vi "Smart Attacker.vi"(8 "error in (no error)":errorcluster, 10 "Map":i32[](array[numeric]), 11 "Mother In":refnum<class "Base Builder.lvclass">) -> (0 "error out":errorcluster, 1 "Direction":T1, 2 "Action":T2, 3 "Mother Out":refnum<class "Base Builder.lvclass">, 4 "Replicated":refnum<class "Square.lvclass">)   [LabVIEW 2015, in "Base Builder.lvclass"]
uses:
  Base Builder/Base Builder.lvclass
  Type Defs/Action Enum.ctl
  Type Defs/Direction Enum.ctl
  Square/Square.lvclass
  Base Builder/Base Builder.lvclass/Base Builder.ctl
  Formics/Attack Options.ctl
  Formics/Coward Options.ctl
  Common/Common.lvlib
  Formics/Formics.lvclass
  Type Defs/SB Type Defs.lvlib
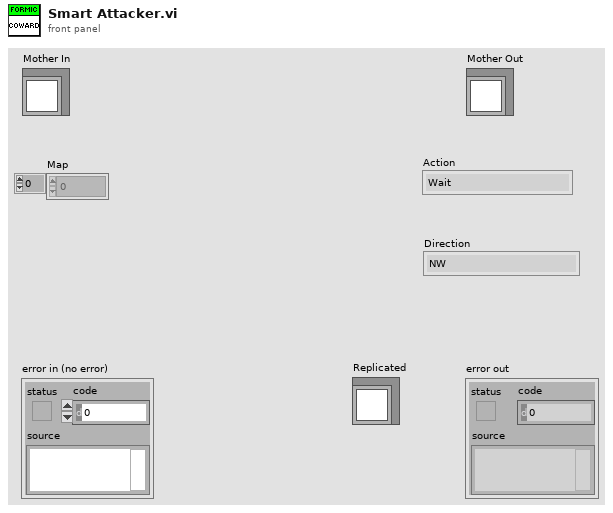
[diagram p1: front panel]
types:
  T1 = typedef "SB Type Defs.lvlib/Direction Enum.ctl" = enum16{"NW", "N", "NE", "E", "SE", "S", "SW", "W"}
  T2 = typedef "SB Type Defs.lvlib/Action Enum.ctl" = enum16{"Wait", "Move", "Attack", "Replicate"}
  T3 = typedef "Formics.lvclass/Coward Options.ctl" = enum16{"Go", "Attack behind and continue", "Attack behind and recheck", "Move Back", "Check if still there"}
  T4 = typedef "Formics.lvclass/Attack Options.ctl" = enum16{"Attack", "Run", "Distract"}
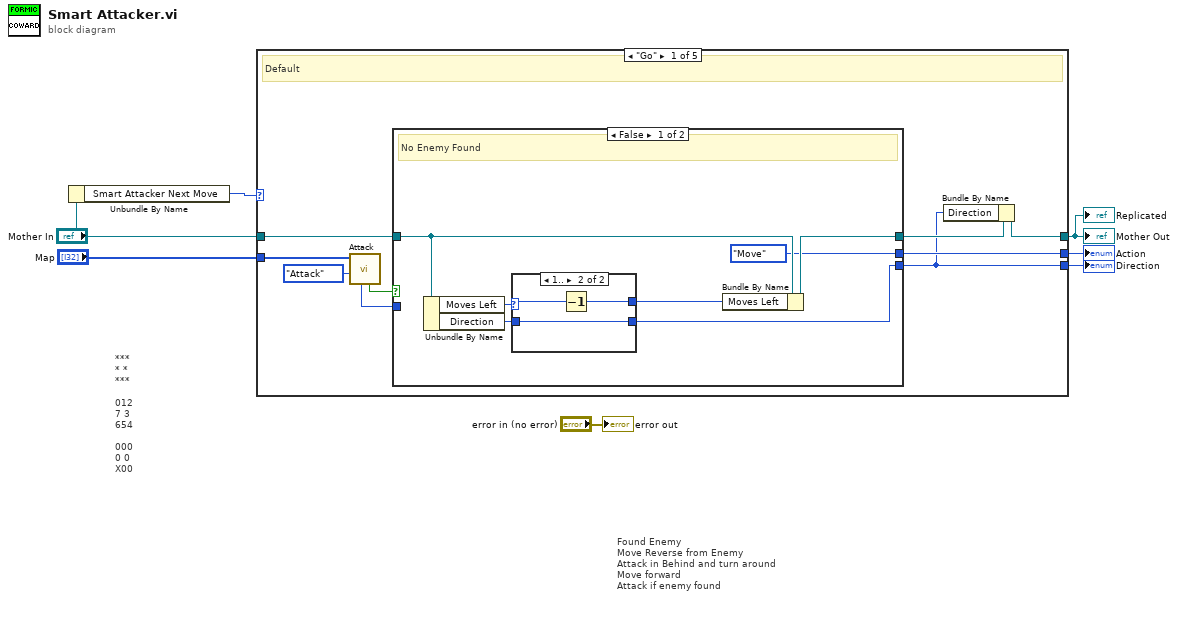
[diagram p0: block diagram]
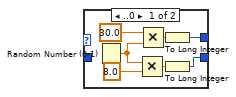
[diagram p2: hidden frame]
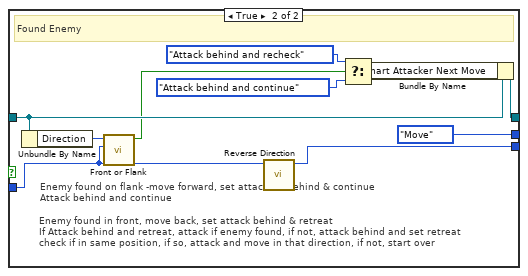
[diagram p3: hidden frame]
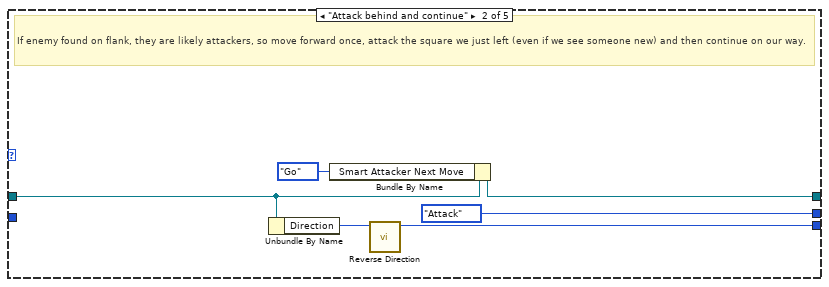
[diagram p4: hidden frame]
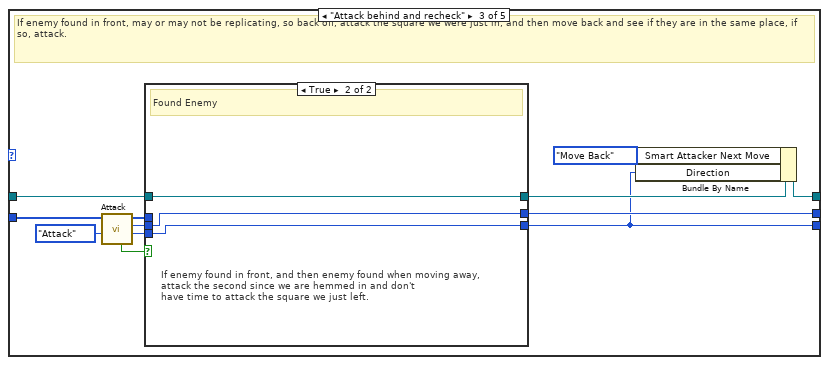
[diagram p5: hidden frame]
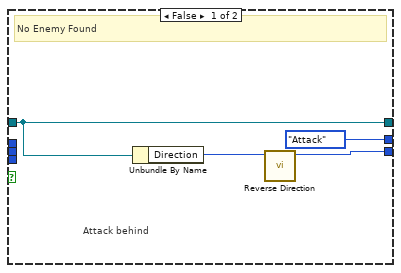
[diagram p6: hidden frame]
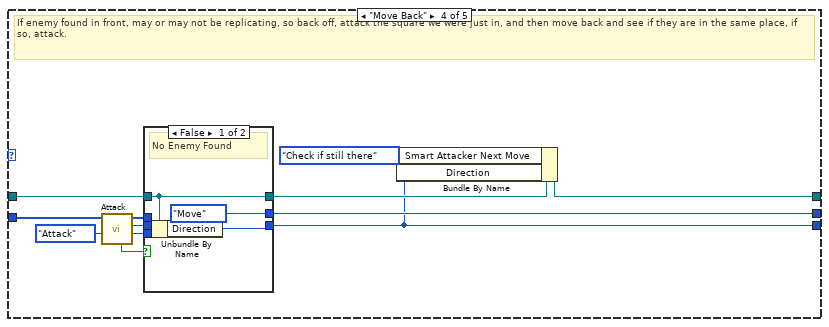
[diagram p7: hidden frame]
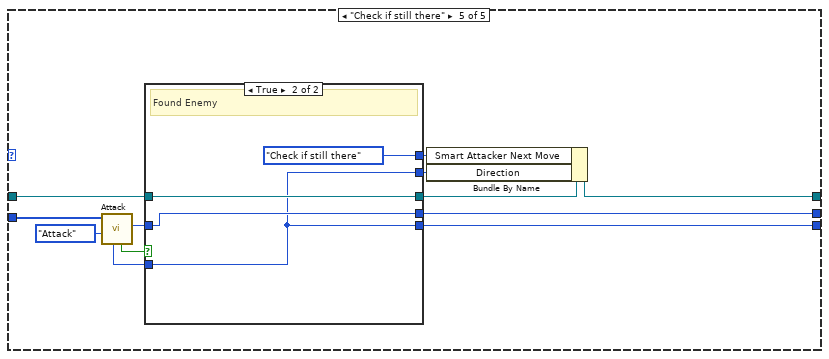
[diagram p9: hidden frame]
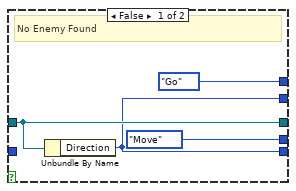
[diagram p10: hidden frame]
diagram:
  # "Found Enemy\nMove Reverse from Enemy\nAttack in Behind and turn around\nMove forward\nAttack if enemy found"
  # "***\n* *\n***\n\n012\n7 3\n654\n\n000\n0 0\nX00"
  n1 = Unbundle By Name("Mother In") -> ("Smart Attacker Next Move"=w2:T3)
  n2 = case shown="\"Go\"" w2 {
    tunnel: [w14 Action_Enum."Attack" ("Action") w58 w77 w95] -> w6
    tunnel: [w9 w48 w50 w69 w94] -> w5
    tunnel: [w10 w47 w52 w71 w90] -> w1
    tunnel: "Map" -> [w12 _ w54 w73 w92]
    tunnel: "Mother In" -> [w11 w44 w53 w72 w91]
    frame "Go" {
      # "Default"
      n3 = call "Attack.vi"("Attack?"=Attack_Options."Attack", "Maze (0: Empty, -1: Enemy. >0: Teammate"=w12) -> ("Enemy Found?"=w15:bool, "Enemy Direction"=w8:i32)  [unwired: 4 in, 4 out]
      n4 = case shown="False" w15 {
        tunnel: [Action_Enum."Move" ("Action") Action_Enum."Move" ("Action")] -> w14
        tunnel: [w17 w35] -> w9
        tunnel: w11 -> [w23 w43]
        tunnel: [w22 w42] -> w13
        tunnel: w8 -> [_ w34]
        frame False {
          # "No Enemy Found"
          n5 = Unbundle By Name(w23) -> ("Moves Left"=w20:u8, "Direction"=w18:T1)
          n6 = case shown="1.." w20 {
            selector: w20 -> [_ w33]
            tunnel: [w25 w32] -> w19
            tunnel: [w24 w31] -> w17
            tunnel: w18 -> [_ w31]
            frame ..0 {
              n7 = Random Number (0-1)() -> (number: 0 to 1=w26:dbl)
              n8 = Multiply(x=w26, y=8.0) -> (x*y=w30:dbl)
              n9 = Multiply(x=30.0 ("t"), y=w26) -> (x*y=w28:dbl)
              n10 = To Long Integer(number=w28) -> (32bit integer=w25:i32)
              n11 = To Long Integer(number=w30) -> (32bit integer=w24:i32)
            }
            frame 1.. {
              n12 = Decrement(x=w33) -> (x-1=w32:u8)
            }
          }
          n13 = Bundle By Name(cluster=w23, "Moves Left"=w19) -> (w22:refnum<class "Base Builder.lvclass">)
        }
        frame True {
          # "Enemy found in front, move back, set attack behind & retreat\nIf Attack behind and retreat, attack if enemy found, if not, attack behind and set retreat\ncheck if in same position, if so, attack and move in that direction, if not, start over"
          # "Enemy found on flank -move forward, set attack for behind & continue\nAttack behind and continue"
          # "Found Enemy"
          n14 = Unbundle By Name(w43) -> ("Direction"=w41:T1)
          n15 = call "Front or Flank.vi"("Enemy Direction"=w34, "Direction"=w41) -> ("Front?"=w40:bool)  [unwired: 9 in]
          n16 = call "Reverse Direction.vi"("Direction"=w34) -> ("Numeric"=w35:i32)  [unwired: 10 in]
          n17 = Select(t=Coward_Options."Attack behind and recheck" ("Next Move"), s=w40, f=Coward_Options."Attack behind and continue" ("Next Move")) -> (s? t:f=w36:T3)
          n18 = Bundle By Name(cluster=w43, "Smart Attacker Next Move"=w36) -> (w42:refnum<class "Base Builder.lvclass">)
        }
      }
      n19 = Bundle By Name(cluster=w13, "Direction"=w9) -> (w10:refnum<class "Base Builder.lvclass">)
    }
    frame "Attack behind and continue" {
      # "If enemy found on flank, they are likely attackers, so move forward once, attack the square we just left (even if we see someone new) and then continue on our way."
      n20 = Unbundle By Name(w44) -> ("Direction"=w46:T1)
      n21 = Bundle By Name(cluster=w44, "Smart Attacker Next Move"=Coward_Options."Go" ("Next Move")) -> (w47:refnum<class "Base Builder.lvclass">)
      n22 = call "Reverse Direction.vi"("Direction"=w46) -> ("Numeric"=w48:i32)  [unwired: 10 in]
    }
    frame "Attack behind and recheck" {
      # "If enemy found in front, may or may not be replicating, so back off, attack the square we were just in, and then move back and see if they are in the same place, if so, attack."
      n23 = call "Attack.vi"("Attack?"=Attack_Options."Attack", "Maze (0: Empty, -1: Enemy. >0: Teammate"=w54) -> ("Direction"=w57:i32, "Action"=w59:T2, "Maze (0: Empty, -1: Enemy. >0: Teammate 2"=w55:i32[], "Enemy Found?"=w60:bool)  [unwired: 4 in, 2 out]
      n24 = case shown="True" w60 {
        tunnel: w59 -> [_ w67]
        tunnel: [Action_Enum."Attack" ("Action") w67] -> w58
        tunnel: w57 -> [_ w66]
        tunnel: [w62 w66] -> w50
        tunnel: w55 -> [_ _]
        tunnel: w53 -> [w64 w68]
        tunnel: [w64 w68] -> w56
        frame False {
          # "Attack behind"
          # "No Enemy Found"
          n25 = Unbundle By Name(w64) -> ("Direction"=w63:T1)
          n26 = call "Reverse Direction.vi"("Direction"=w63) -> ("Numeric"=w62:i32)  [unwired: 10 in]
        }
        frame True {
          # "If enemy found in front, and then enemy found when moving away, \nattack the second since we are hemmed in and don't \nhave time to attack the square we just left."
          # "Found Enemy"
        }
      }
      n27 = Bundle By Name(cluster=w56, "Smart Attacker Next Move"=Coward_Options."Move Back" ("Next Move"), "Direction"=w50) -> (w52:refnum<class "Base Builder.lvclass">)
    }
    frame "Move Back" {
      # "If enemy found in front, may or may not be replicating, so back off, attack the square we were just in, and then move back and see if they are in the same place, if so, attack."
      n28 = call "Attack.vi"("Attack?"=Attack_Options."Attack", "Maze (0: Empty, -1: Enemy. >0: Teammate"=w73) -> ("Direction"=w76:i32, "Action"=w78:T2, "Maze (0: Empty, -1: Enemy. >0: Teammate 2"=w74:i32[], "Enemy Found?"=w79:bool)  [unwired: 4 in, 2 out]
      n29 = case shown="False" w79 {
        tunnel: w78 -> [_ w85]
        tunnel: [Action_Enum."Move" ("Action") w85] -> w77
        tunnel: w76 -> [_ w84]
        tunnel: [w81 w84] -> w69
        tunnel: w74 -> [_ _]
        tunnel: w72 -> [w82 w86]
        tunnel: [w82 w86] -> w75
        frame False {
          # "No Enemy Found"
          n30 = Unbundle By Name(w82) -> ("Direction"=w81:T1)
        }
        frame True {
          # "If enemy appears, attack it."
          # "Found Enemy"
        }
      }
      n31 = Bundle By Name(cluster=w75, "Smart Attacker Next Move"=Coward_Options."Check if still there" ("Next Move"), "Direction"=w69) -> (w71:refnum<class "Base Builder.lvclass">)
    }
    frame "Check if still there" {
      n32 = call "Attack.vi"("Attack?"=Attack_Options."Attack", "Maze (0: Empty, -1: Enemy. >0: Teammate"=w92) -> ("Action"=w96:T2, "Enemy Found?"=w97:bool, "Enemy Direction"=w87:i32)  [unwired: 4 in, 3 out]
      n33 = case shown="True" w97 {
        tunnel: w96 -> [_ w104]
        tunnel: [Action_Enum."Move" ("Action") w104] -> w95
        tunnel: [w100 w103] -> w94
        tunnel: w91 -> [w101 w106]
        tunnel: [w101 w106] -> w93
        tunnel: [w100 w103] -> w89
        tunnel: [Coward_Options."Go" ("Next Move") Coward_Options."Check if still there" ("Next Move")] -> w88
        tunnel: w87 -> [_ w103]
        frame False {
          # "No Enemy Found"
          n34 = Unbundle By Name(w101) -> ("Direction"=w100:T1)
        }
        frame True {
          # "Found Enemy"
        }
      }
      n35 = Bundle By Name(cluster=w93, "Smart Attacker Next Move"=w88, "Direction"=w89) -> (w90:refnum<class "Base Builder.lvclass">)
    }
  }
  "Mother Out" <- w1
  "Action" <- w6
  "Direction" <- w5
  "Replicated" <- w1
  "error out" <- "error in (no error)"
